vi "Generate Piece.vi"(8 "error in (no error)":errorcluster caption="entrée d'erreur (pas d'erreur)", 11 "Game Board en entrée":refnum<class "Game Board.lvclass">) -> (0 "error out":errorcluster caption="sortie d'erreur", 3 "Game Board en sortie":refnum<class "Game Board.lvclass">)   [LabVIEW 2017, in "Game Board.lvclass"]
uses:
  Game Board.lvclass
  Game Board.lvclass/Game Board.ctl
  Piece of Bricks_class/Piece of Bricks.lvclass
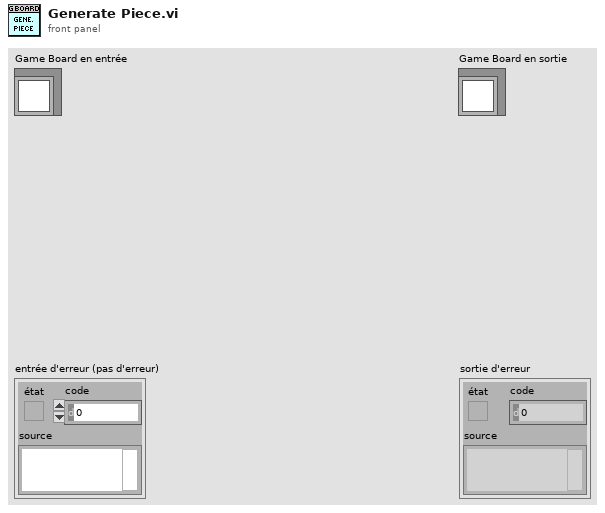
[diagram p1: front panel]
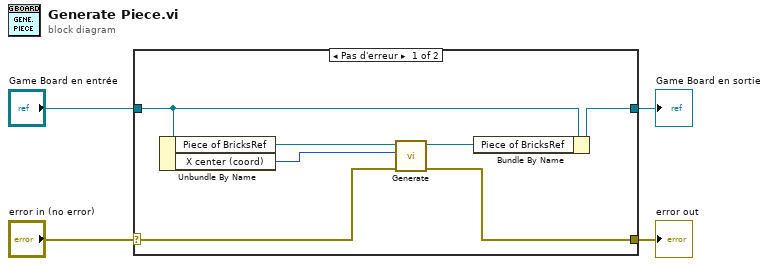
[diagram p0: block diagram]
diagram:
  n1 = case shown="Pas d'erreur" "error in (no error)" {
    selector: "error in (no error)" -> [w6 w13]
    tunnel: [w5 w13] -> w3
    tunnel: [w10 w12] -> w1
    tunnel: "Game Board en entrée" -> [w11 w12]
    frame No Error {
      n2 = Unbundle By Name(w11) -> ("Piece of BricksRef"=w9:refnum<class "Piece of Bricks.lvclass">, "X center (coord)"=w8:i32)
      n3 = call-dynamic "Generate.vi"("error in (no error)"=w6, "X Center"=w8, "object in"=w9) -> ("error out"=w5:errorcluster, "object out"=w7:refnum<class "Piece of Bricks.lvclass">)  [unwired: 7 in]
      n4 = Bundle By Name(cluster=w11, "Piece of BricksRef"=w7) -> (w10:refnum<class "Game Board.lvclass">)
    }
    frame Error {
    }
  }
  "error out" <- w3
  "Game Board en sortie" <- w1
